vi "Mathematics_G0conversion.vi"(5 "Bias (0.2) / V":dbl=0.2, 6 "Amplification (1E6) / V/A":dbl=1000000.0, 8 "Error In":errorcluster, 11 "Femto Output (0) / V":dbl) -> (0 "Error Out":errorcluster, 3 "G/G0":dbl)   [LabVIEW 2023]
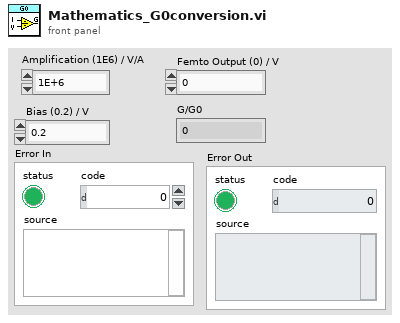
[diagram p1: front panel]
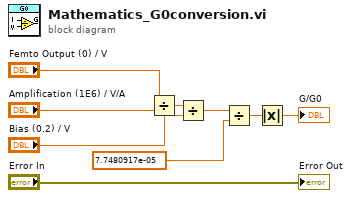
[diagram p0: block diagram]
diagram:
  n1 = Divide(x="Femto Output (0) / V", y="Amplification (1E6) / V/A") -> (x/y=w8:dbl)
  n2 = Divide(x=w8, y="Bias (0.2) / V") -> (x/y=w9:dbl)
  n3 = Divide(x=w9, y=7.7480917e-05) -> (x/y=w5:dbl)
  n4 = Absolute Value(x=w5) -> (abs(x)=→"G/G0":dbl)
  "Error Out" <- "Error In"
